vi "Load Stocks.vi"(7 "Use Default libelle path ? (Y)":bool=TRUE, 9 "file path (dialog if empty)":path caption="chemin du fichier (boîte de dialogue si vide)", 10 "Symbol_Suffix (.PA)":string=".PA", 11 "Currency (Euro)":T1 items=["Euro", "Dollar", "Yen", "RIM", "CHF"]) -> (1 "Count":i32, 2 "Stocks":refnum<class "Stock.lvclass">[](array[class]))   [LabVIEW 2012]
uses:
  controls/Currencies.ctl
  Stock/Stock.lvclass
  Stock/Stock.lvclass/Stock.ctl
  <vilib>/Utility/file.llb/Read From Spreadsheet File (string).vi
panel:
  out "all rows":string[][](array[string]) caption="toutes les lignes"
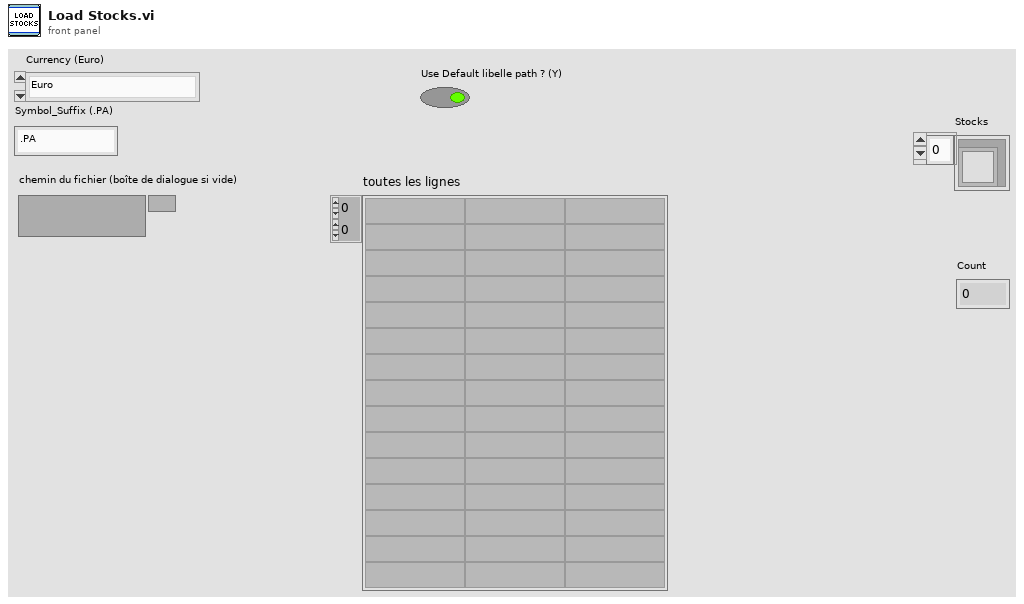
[diagram p1: front panel]
types:
  T1 = typedef "Currencies.ctl" = u16
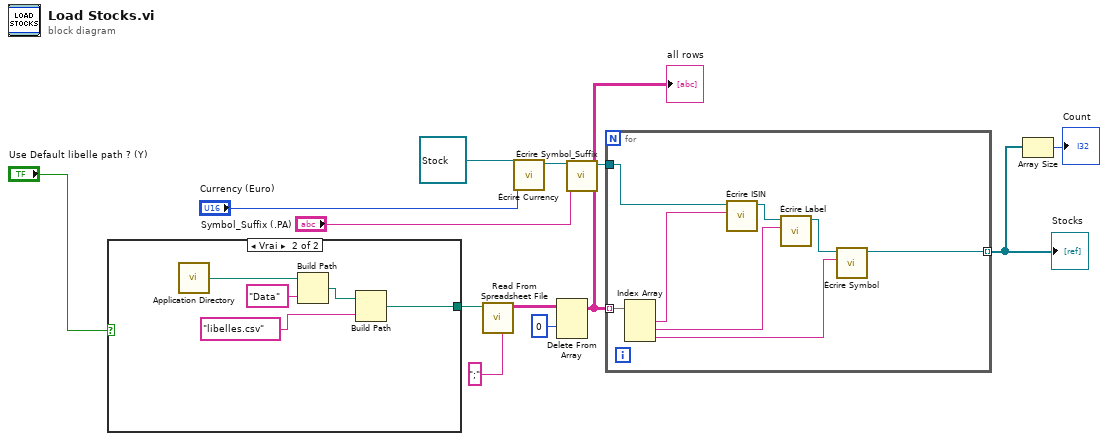
[diagram p0: block diagram]
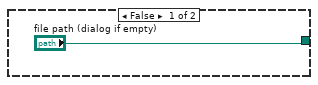
[diagram p2: hidden frame]
diagram:
  n1 = case shown="Vrai" "Use Default libelle path ? (Y)" {
    tunnel: ["file path (dialog if empty)" w15] -> w12
    frame False {
    }
    frame True {
      n2 = call <vilib>:"Application Directory.vi"() -> ("Application Directory"=w19:path)
      n3 = Build Path(base path=w19, name or relative path="Data" ("nom ou chemin relatif")) -> (appended path=w17:path)
      n4 = Build Path(base path=w17, name or relative path="libelles.csv" ("nom ou chemin relatif")) -> (appended path=w15:path)
    }
  }
  n5 = call-poly <vilib>:"Read From Spreadsheet File.vi"("delimiter (\\t)"=";" ("delimiter (\\t)"), "file path (dialog if empty)"=w12) -> ("all rows"=w10:string[][])  [unwired: 5 in, 4 out]
  n6 = call "Écrire Currency.vi"("Currency"="Currency (Euro)", "Share en entrée"=refnum<class "Stock.lvclass"> refnum ("Stock.lvclass")) -> ("Share en sortie"=w5:refnum<class "Stock.lvclass">)  [unwired: 8 in, 1 out]
  n7 = Delete From Array(array=w10, index (row)=0 ("indice (ligne)")) -> (array with subset deleted=w8:string[][])  [unwired: 2 in, 1 out]
  "all rows" <- w8
  n8 = call "Écrire Symbol_Suffix.vi"("Symbol_Suffix"="Symbol_Suffix (.PA)", "Stock en entrée"=w5) -> ("Stock en sortie"=w4:refnum<class "Stock.lvclass">)  [unwired: 8 in, 1 out]
  n9 = for {
    tunnel: w8 -> [w27] mode=indexing
    tunnel: w4 -> [w26]
    tunnel: [w20] -> w2 mode=indexing
    n10 = Index Array(array=w27) -> (element #1=w25:string, element #2=w23:string, element #3=w21:string)  [unwired: 3 in]
    n11 = call "Écrire ISIN.vi"("ISIN"=w25, "Share en entrée"=w26) -> ("Share en sortie"=w24:refnum<class "Stock.lvclass">)  [unwired: 8 in, 1 out]
    n12 = call "Écrire Label.vi"("Label"=w23, "Share en entrée"=w24) -> ("Share en sortie"=w22:refnum<class "Stock.lvclass">)  [unwired: 8 in, 1 out]
    n13 = call "Écrire Symbol.vi"("Symbol"=w21, "Share en entrée"=w22) -> ("Share en sortie"=w20:refnum<class "Stock.lvclass">)  [unwired: 8 in, 1 out]
  }
  "Stocks" <- w2
  n14 = Array Size(array=w2) -> (size(s)=→"Count":i32)
